vi "Static dual axis example.vi"   [LabVIEW 2019]
uses:
  Axis Manager/Axis config.ctl
  Axis Manager/Axis enum.ctl
panel:
  # "MAIN Example\n\nOpen Block Diagram (ctrl-E)\nto see the code."
types:
  T1 = typedef "Axis config.ctl" = cluster{"Letter":string, "Stagetype":T2}
  T2 = typedef "Axis enum.ctl" = enum16{"XLA with 50 µm resolution", "XLA with 10 µm resolution", "XLA with 1250 nm resolution", "XLA with 312 nm resolution", "XLA with 78 nm resolution", "XLS with 1250 nm resolution", "XLS with 312 nm resolution", "XLS with 78nm resolution", "XLS with 5nm resolution", "XLS with 1 nm resolution", "XRT-A with 109 µrad resolution", "XRT-U-30 with 109 µrad resolution", "XRT-U-30 with 49 µrad resolution", "XRT-U-30 with 19 µrad resolution", "XRT-U-30 with 3 µrad resolution", "XRT-U-40 with 109 µrad resolution", "XRT-U 40 with 49 µrad resolution", "XRT-U-40 with 19 µrad resolution", "XRT-U-40 with 3 µrad resolution", "XRT-U-60 with 109 µrad resolution", "XRT-U-60 with 49 µrad resolution", "XRT-U-60 with 19 µrad resolution", "XRT-U-60 with 3 µrad resolution"}
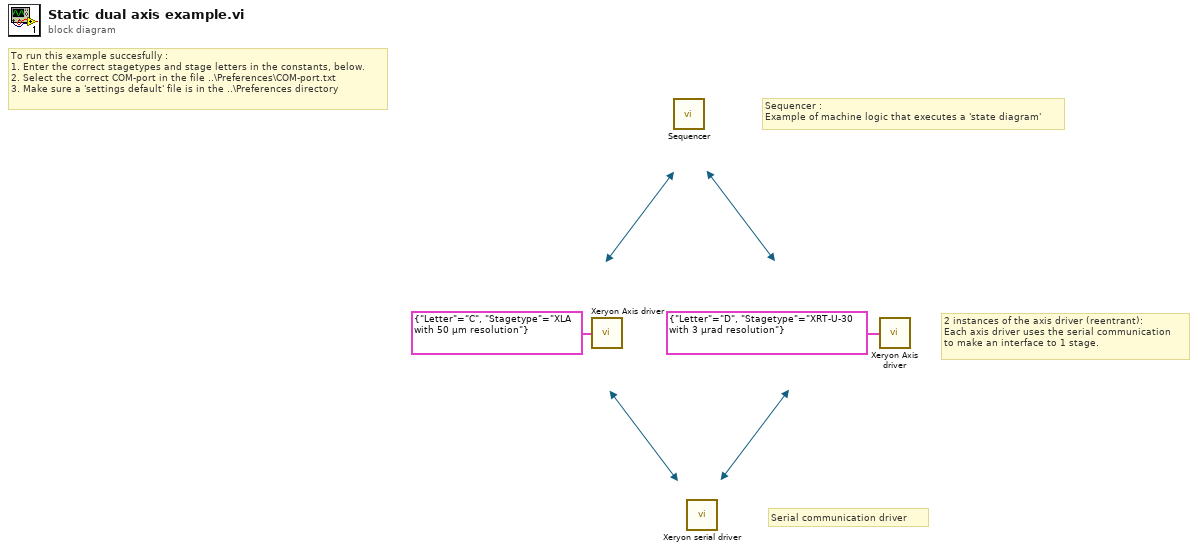
[diagram p0: block diagram]
diagram:
  # "To run this example succesfully :\n1. Enter the correct stagetypes and stage letters in the constants, below.\n2. Select the correct COM-port in the file ..\\Preferences\\COM-port.txt\n3. Make sure a 'settings default' file is in the ..\\Preferences directory"
  # "Sequencer :\nExample of machine logic that executes a 'state diagram'"
  # "2 instances of the axis driver (reentrant):\nEach axis driver uses the serial communication\nto make an interface to 1 stage."
  # "Serial communication driver"
  n1 = call "Xeryon Axis driver.vi"("Config"=T1 {"Letter"="C", "Stagetype"=enum."XLA with 50 µm resolution"}) -> ()  [unwired: 5 in]
  n2 = call "Sequencer.vi"() -> ()  [unwired: 12 in]
  n3 = call "Xeryon serial driver.vi"() -> ()  [unwired: 6 in]
  n4 = call "Xeryon Axis driver.vi"("Config"=T1 {"Letter"="D", "Stagetype"=enum."XRT-U-30 with 3 µrad resolution"}) -> ()  [unwired: 5 in]
